vi "Search Element By Tag.vi"(8 "Error In":errorcluster, 10 "Element Tag":string, 11 "Display Manager In":refnum<class "Display Manager.lvclass">) -> (0 "Error Out":errorcluster, 1 "Found?":bool, 2 "Display Element":refnum<class "Display Element.lvclass">, 3 "Display Manager Out":refnum<class "Display Manager.lvclass">)   [LabVIEW 2021, in "Display Manager.lvclass"]
uses:
  Display Manager.lvclass
  Display Element/Display Element.lvclass
  Accessors/Display Elements/Get Display Elements.vi
  <vilib>/Utility/error.llb/Error Cluster From Error Code.vi
  <vilib>/ErrorRing/Error Ring.xnode
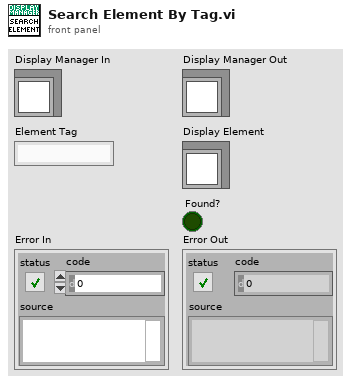
[diagram p1: front panel]
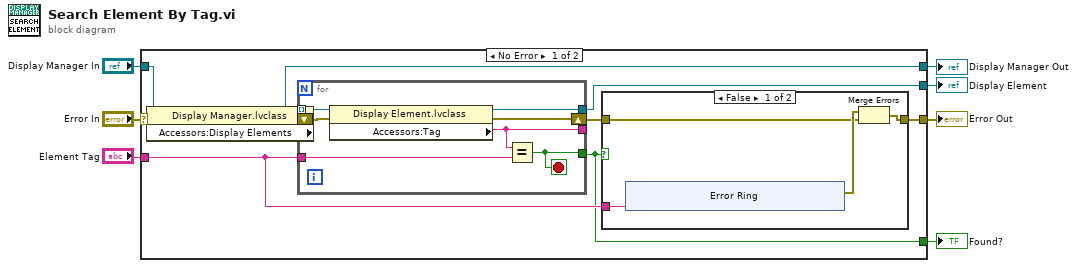
[diagram p0: block diagram]
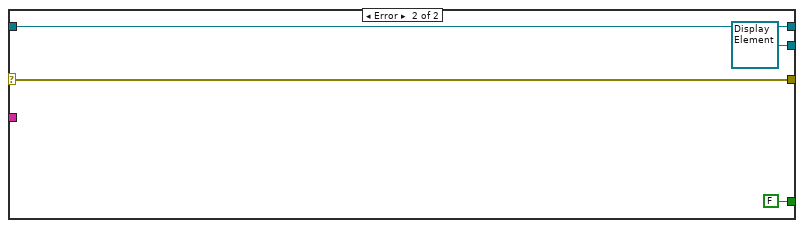
[diagram p3: hidden frame]
diagram:
  n1 = case shown="No Error" "Error In" {
    selector: "Error In" -> [w16 w39]
    tunnel: "Display Manager In" -> [w17 w40]
    tunnel: [w15 w40] -> w5
    tunnel: [w9 w39] -> w4
    tunnel: "Element Tag" -> [w10 _]
    tunnel: [w12 refnum<class "Display Element.lvclass"> refnum ("Display Element.lvclass")] -> w2
    tunnel: [w8 FALSE] -> w1
    frame No Error {
      n2 = property class="Display Manager.lvclass"(reference=w17, error in=w16) -> (reference out=w15:refnum<class "Display Manager.lvclass">, error out=w13:errorcluster, "Accessors:Display Elements"=w14:refnum<class "Display Element.lvclass">[])
      n3 = for {
        tunnel: w14 -> [w24] mode=indexing
        tunnel: [w20] -> _
        shift-right: [w21] -> w11
        shift-left: w13 -> [w23]
        tunnel: [w22] -> w12
        tunnel: w10 -> [w19]
        tunnel: [w18] -> w8
        stop <- w18 stop-if-true
        n4 = property class="Display Element.lvclass"(reference=w24, error in=w23) -> (reference out=w22:refnum<class "Display Element.lvclass">, error out=w21:errorcluster, "Accessors:Tag"=w20:string)
        n5 = Equal?(x=w20, y=w19) -> (x = y?=w18:bool)
      }
      n6 = case shown="False" w8 {
        tunnel: w11 -> [w26 w36]
        tunnel: w10 -> [w28 _]
        tunnel: [w25 w36] -> w9
        frame False {
          n7 = xnode "Error Ring"("parameter 0"=w28) -> ("error out"=w27:errorcluster)
          n8 = Merge Errors(w27, w26) -> (w25:errorcluster)
        }
        frame True {
        }
      }
    }
    frame Error {
    }
  }
  "Display Manager Out" <- w5
  "Error Out" <- w4
  "Display Element" <- w2
  "Found?" <- w1
